vi "spliteFTPpathLeaf.vi"(11 "Name":string) -> (3 "String":string)   [LabVIEW 2017, in "_Try Beta Version of CSMF.lvlib"]
uses:
  _Try Beta Version of CSMF.lvlib
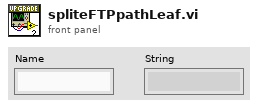
[diagram p1: front panel]
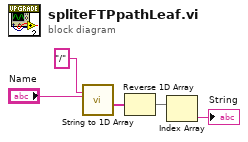
[diagram p0: block diagram]
diagram:
  n1 = call "String to 1D Array.vi"("delimiter (Tab)"="/", "string"="Name") -> ("Array of Strings"=w4:string[])  [unwired: 9 in]
  n2 = Reverse 1D Array(array=w4) -> (reversed array=w3:string[])
  n3 = Index Array(array=w3) -> (element=→"String":string)  [unwired: 1 in]
